vi "Graph Screen.vi"() -> ()   [LabVIEW 2022 SP3]
uses:
  <vilib>/numeric/Random Number (Range) U64.vi
  <vilib>/numeric/sub_Random U32.vi
panel:
  out "Waveform 6":u64[][](graph)
  out "Waveform 5":u64[][](graph)
  out "Waveform 4":u64[][](graph)
  out "Waveform 3":u64[][](graph)
  out "Waveform 2":u64[][](graph)
  out "Waveform 1":u64[][](graph)
  in  "EXIT":bool
  # "GRAPH SCREEN"
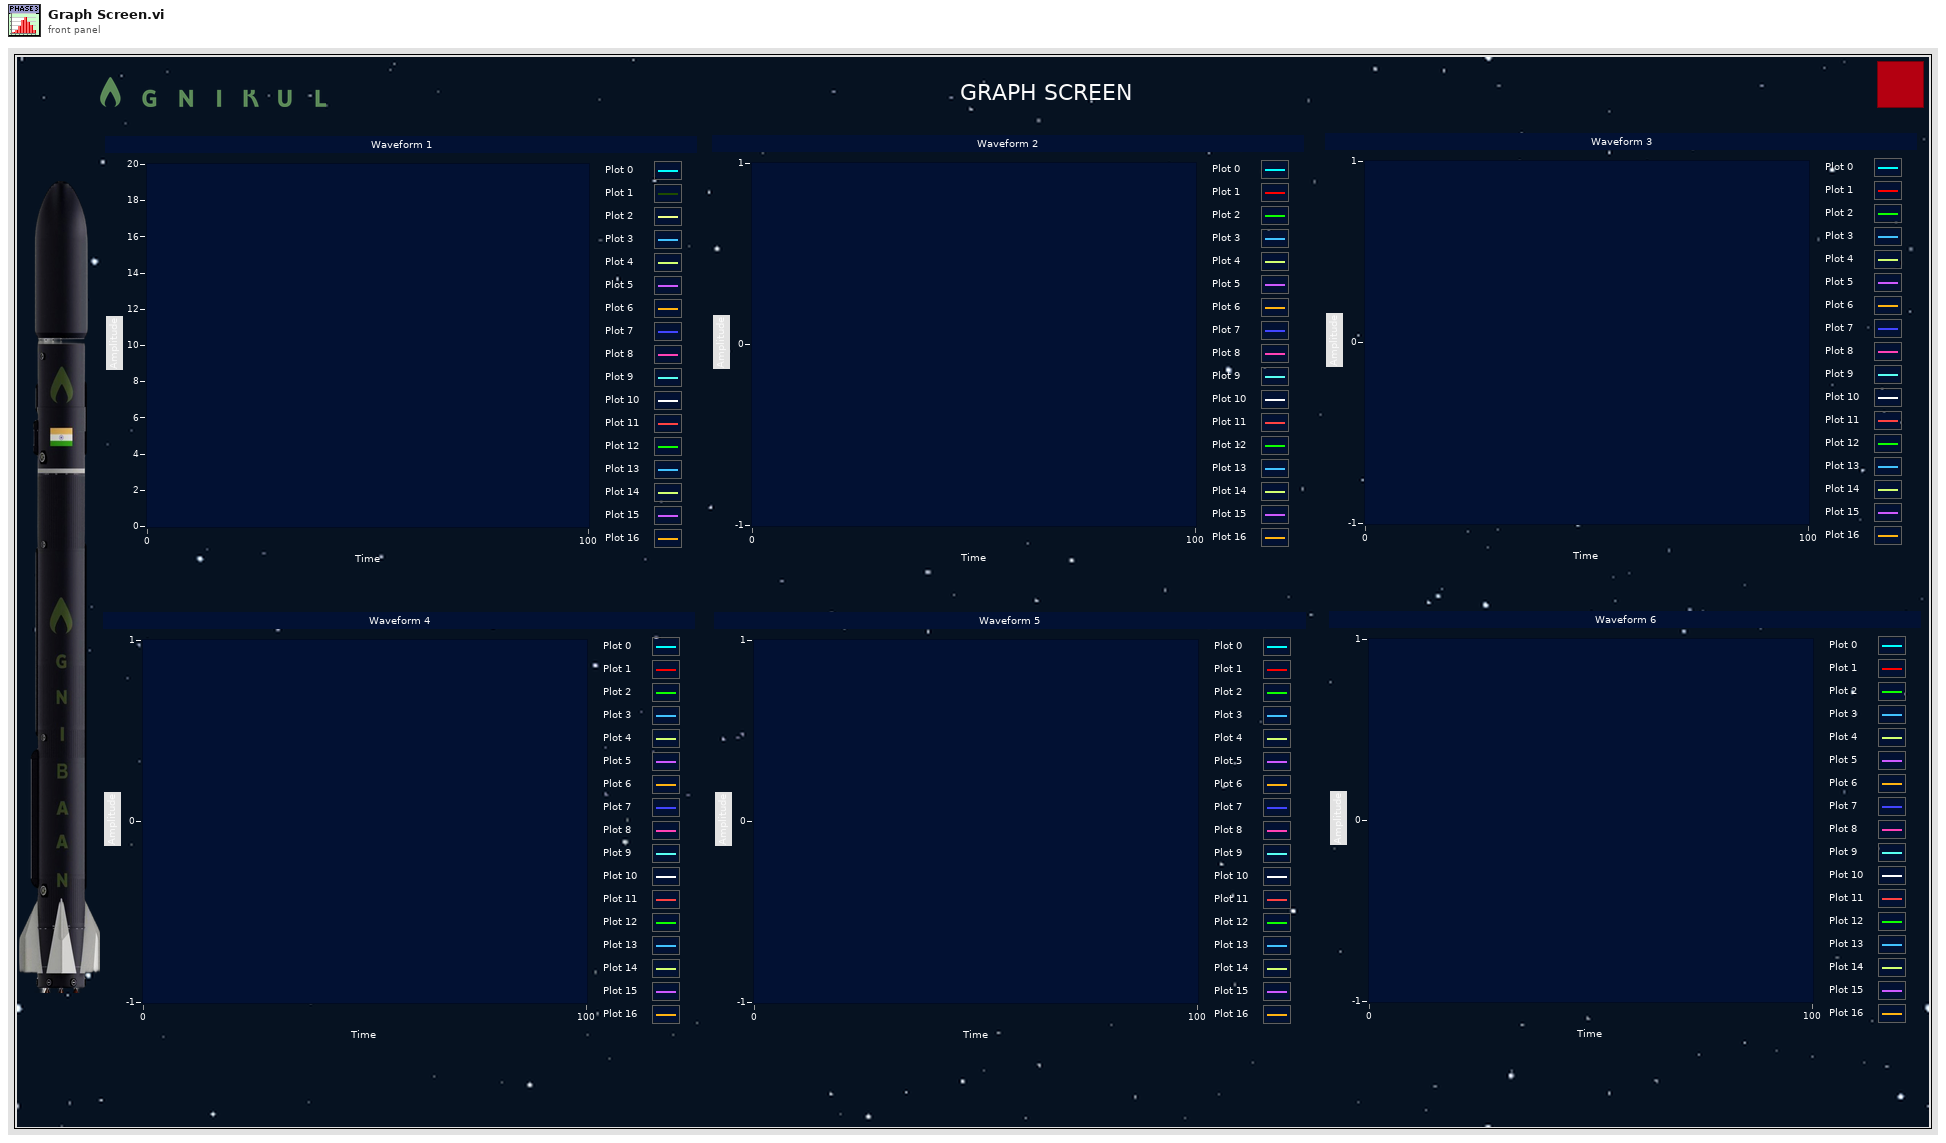
[diagram p1: front panel]
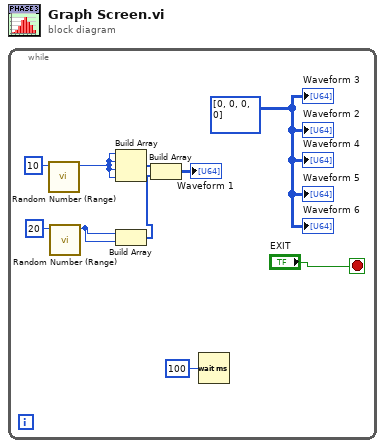
[diagram p0: block diagram]
diagram:
  n1 = while {
    stop <- "EXIT" stop-if-true
    w5 = u64[][] [[0, 0, 0, 0]] ("Waveform 4")
    n2 = call-poly <vilib>:"Random Number (Range).vi"("upper bound (100)"=u64 10) -> ("number"=w6:u64)  [unwired: 10 in]
    n3 = call-poly <vilib>:"Random Number (Range).vi"("upper bound (100)"=u64 20) -> ("number"=w2:u64)  [unwired: 10 in]
    n4 = Build Array(w6, w6, w6, w6) -> (w4:u64[])
    n5 = Build Array(w2, w2) -> (w1:u64[])
    n6 = Build Array(w4, w1) -> (→"Waveform 1":u64[][])
    n7 = Wait (ms)(milliseconds to wait=u32 100) -> ()  [unwired: 1 out]
    "Waveform 2" <- w5
    "Waveform 3" <- w5
    "Waveform 4" <- w5
    "Waveform 5" <- w5
    "Waveform 6" <- w5
  }
